vi "PMS7003_read_v2_subVi.vi"(8 "error in (no error)":errorcluster, 10 "UART connected":bool, 11 "VISA Refnum in":refnum<visa-resource-name>) -> (0 "error out":errorcluster, 1 "Boolean":bool, 2 "VISA Refnum out":refnum<visa-resource-name>, 3 "output cluster":cluster{"PM1.0":i32, "PM2.5":i32, "PM10":i32})   [LabVIEW 2019]
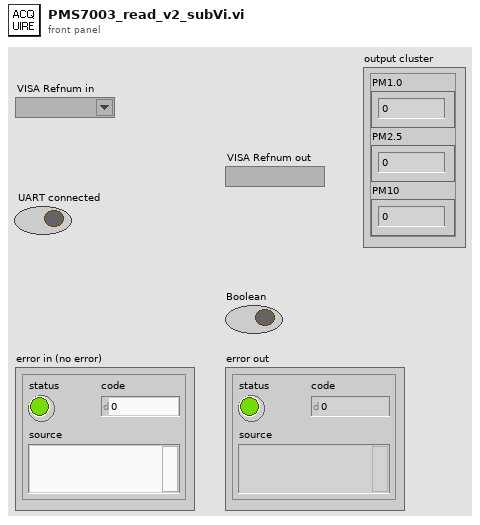
[diagram p1: front panel]
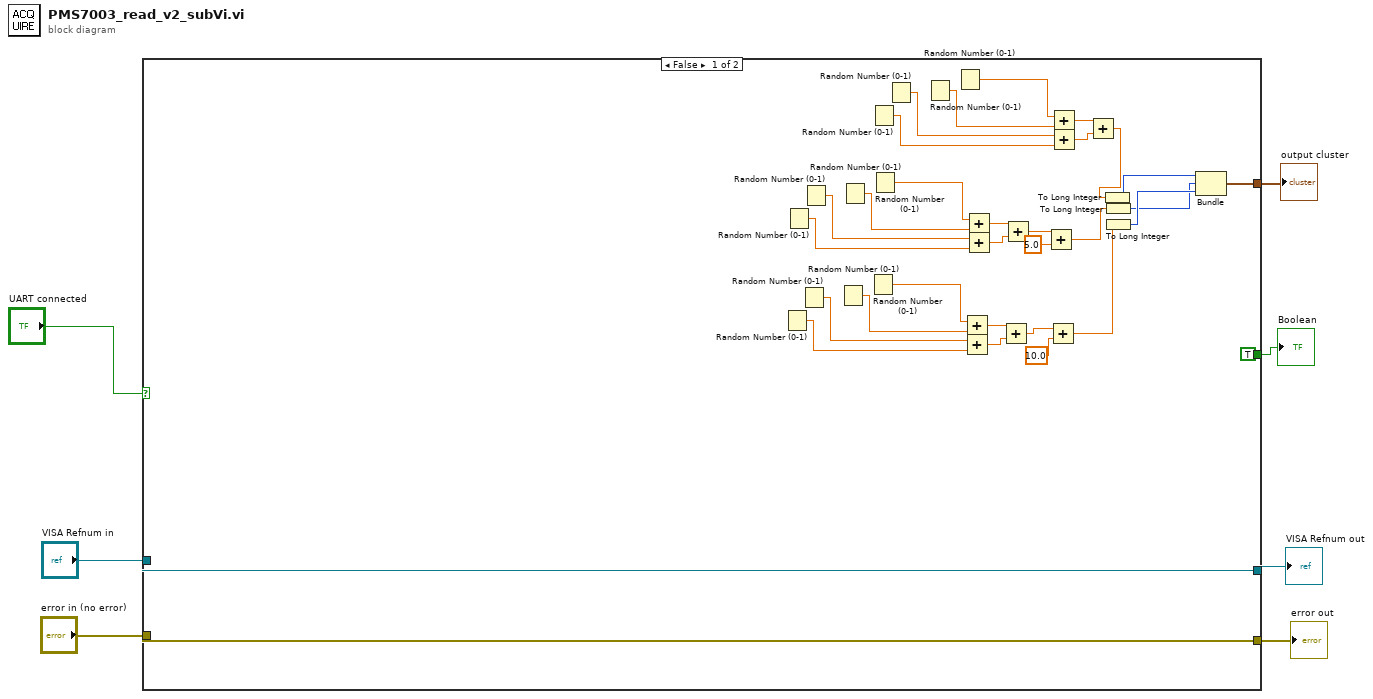
[diagram p0: block diagram]
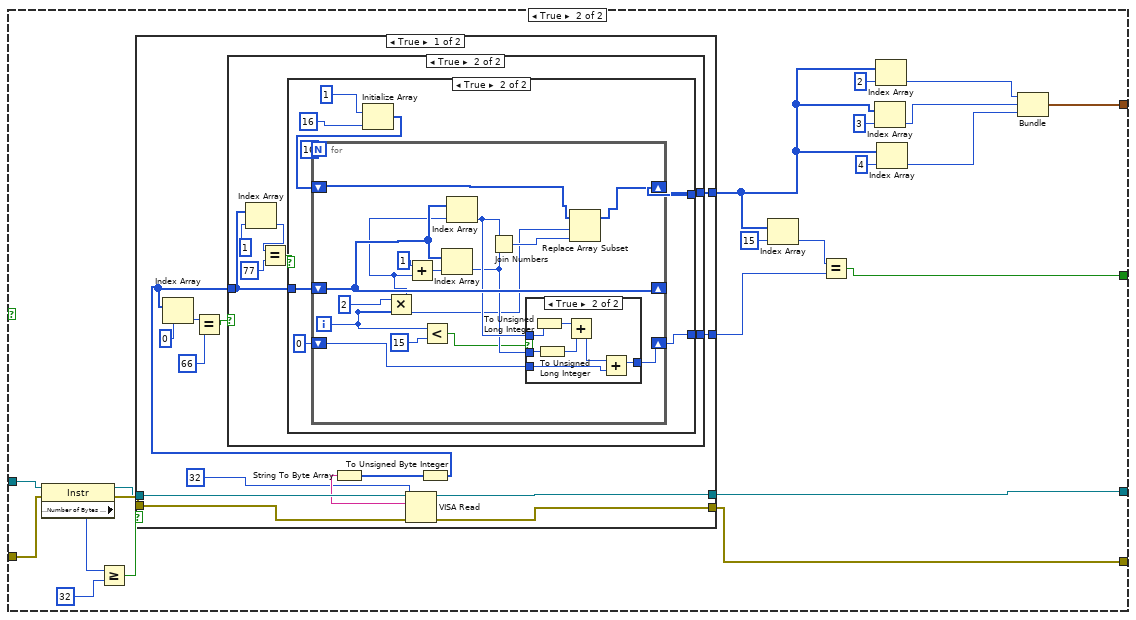
[diagram p2: hidden frame]
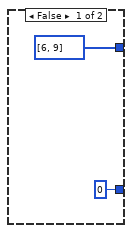
[diagram p3: hidden frame]
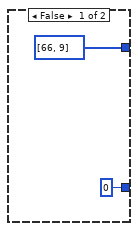
[diagram p4: hidden frame]
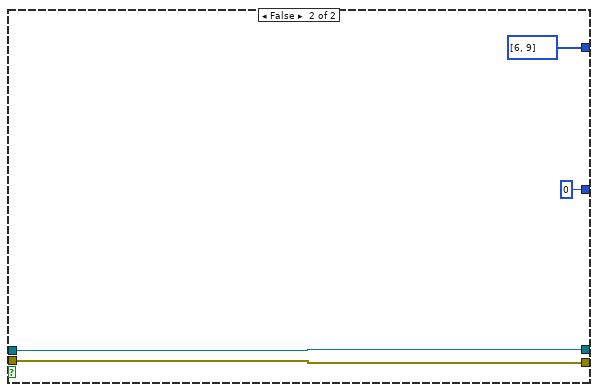
[diagram p6: hidden frame]
diagram:
  n1 = case shown="False" "UART connected" {
    tunnel: "error in (no error)" -> [w38 w59]
    tunnel: "VISA Refnum in" -> [w39 w58]
    tunnel: [TRUE w50] -> w5
    tunnel: [w39 w49] -> w3
    tunnel: [w30 w41] -> w2
    tunnel: [w38 w40] -> w1
    frame False {
      n2 = Random Number (0-1)() -> (number: 0 to 1=w20:dbl)
      n3 = Random Number (0-1)() -> (number: 0 to 1=w26:dbl)
      n4 = Random Number (0-1)() -> (number: 0 to 1=w21:dbl)
      n5 = Random Number (0-1)() -> (number: 0 to 1=w27:dbl)
      n6 = Random Number (0-1)() -> (number: 0 to 1=w22:dbl)
      n7 = Random Number (0-1)() -> (number: 0 to 1=w28:dbl)
      n8 = Random Number (0-1)() -> (number: 0 to 1=w23:dbl)
      n9 = Random Number (0-1)() -> (number: 0 to 1=w33:dbl)
      n10 = Random Number (0-1)() -> (number: 0 to 1=w29:dbl)
      n11 = Random Number (0-1)() -> (number: 0 to 1=w34:dbl)
      n12 = Random Number (0-1)() -> (number: 0 to 1=w35:dbl)
      n13 = Random Number (0-1)() -> (number: 0 to 1=w36:dbl)
      n14 = Add(x=w23, y=w22) -> (x+y=w19:dbl)
      n15 = Add(x=w21, y=w20) -> (x+y=w18:dbl)
      n16 = Add(x=w29, y=w28) -> (x+y=w25:dbl)
      n17 = Add(x=w27, y=w26) -> (x+y=w24:dbl)
      n18 = Add(x=w19, y=w18) -> (x+y=w10:dbl)
      n19 = Add(x=w25, y=w24) -> (x+y=w13:dbl)
      n20 = Add(x=w13, y=5.0) -> (x+y=w11:dbl)
      n21 = Add(x=w10, y=10.0) -> (x+y=w8:dbl)
      n22 = Add(x=w36, y=w35) -> (x+y=w32:dbl)
      n23 = Add(x=w34, y=w33) -> (x+y=w31:dbl)
      n24 = Add(x=w32, y=w31) -> (x+y=w17:dbl)
      n25 = To Long Integer(number=w17) -> (32bit integer=w14:i32)
      n26 = To Long Integer(number=w11) -> (32bit integer=w15:i32)
      n27 = To Long Integer(number=w8) -> (32bit integer=w16:i32)
      n28 = Bundle(w14, w15, w16) -> (w30:cluster{i32, i32, i32})  [unwired: 1 in]
    }
    frame True {
      n29 = property class="Instr"(reference=w58, error in=w59) -> (reference out=w54:refnum<visa-resource-name>, error out=w55:errorcluster, "Serial Settings:Number of Bytes at Serial Port"=w60:u32)
      n30 = Greater Or Equal?(x=w60, y=u32 32) -> (x >= y?=w57:bool)
      n31 = case shown="True" w57 {
        tunnel: [w72 w120] -> w49
        tunnel: w54 -> [w74 w120]
        tunnel: [w71 w119] -> w40
        tunnel: w55 -> [w73 w119]
        tunnel: [w68 u16[] [6, 9]] -> w48
        tunnel: [w62 u32 0] -> w52
        frame True {
          n32 = VISA Read(VISA resource name=w74, byte count=u32 32 ("Read Count 2"), error in (no error)=w73) -> (VISA resource name out=w72:refnum<visa-resource-name>, read buffer=w70:string, error out=w71:errorcluster)  [unwired: 1 out]
          n33 = String To Byte Array(string=w70) -> (unsigned byte array=w69:u8[])
          n34 = To Unsigned Byte Integer(number=w69) -> (unsigned 8bit integer=w63:u8[])
          n35 = Index Array(array=w63, index=0) -> (element=w66:u8)
          n36 = Equal?(x=w66, y=u8 66) -> (x = y?=w64:bool)
          n37 = case shown="True" w64 {
            tunnel: w63 -> [_ w82]
            tunnel: [u16[] [6, 9] w83] -> w68
            tunnel: [u32 0 w77] -> w62
            frame False {
            }
            frame True {
              n38 = Index Array(array=w82, index=1) -> (element=w79:u8)
              n39 = Equal?(x=w79, y=u8 77) -> (x = y?=w78:bool)
              n40 = case shown="True" w78 {
                tunnel: w82 -> [_ w93]
                tunnel: [u16[] [66, 9] w91] -> w83
                tunnel: [u32 0 w87] -> w77
                frame False {
                }
                frame True {
                  n41 = Initialize Array(1 ("index"), 16 ("index")) -> (w90:i32[])
                  n42 = for {
                    N: 16 -> [_]
                    shift-right: [w108] -> _
                    shift-left: w93 -> [w108]
                    shift-right: [w103] -> w91
                    shift-left: w90 -> [w104]
                    shift-right: [w100] -> w87
                    shift-left: u32 0 -> [w96]
                    i -> [w98]
                    n43 = Multiply(x=2, y=w98) -> (x*y=w94:i32)
                    n44 = Add(x=1, y=w94) -> (x+y=w95:i32)
                    n45 = Less?(x=w98, y=15) -> (x < y?=w99:bool)
                    n46 = Index Array(array=w108, index=w95) -> (element=w101:u8)
                    n47 = Index Array(array=w108, index=w94) -> (element=w102:u8)
                    n48 = Join Numbers(hi=w102, lo=w101) -> ((hi.lo)=w105:u16)
                    n49 = case shown="True" w99 {
                      tunnel: w102 -> [_ w112]
                      tunnel: w101 -> [_ w111]
                      tunnel: [w109 w115] -> w100
                      tunnel: w96 -> [w109 w110]
                      frame False {
                      }
                      frame True {
                        n50 = To Unsigned Long Integer(number=w112) -> (unsigned 32bit integer=w113:u32)
                        n51 = To Unsigned Long Integer(number=w111) -> (unsigned 32bit integer=w114:u32)
                        n52 = Add(x=w113, y=w114) -> (x+y=w116:u32)
                        n53 = Add(x=w116, y=w110) -> (x+y=w115:u32)
                      }
                    }
                    n54 = Replace Array Subset(array=w104, new element=w105, index=w98) -> (w103:i32[])
                  }
                }
              }
            }
          }
        }
        frame False {
        }
      }
      n55 = Index Array(array=w48, index=15) -> (element=w53:i32)
      n56 = Equal?(x=w53, y=w52) -> (x = y?=w50:bool)
      n57 = Index Array(array=w48, index=3) -> (element=w43:i32)
      n58 = Index Array(array=w48, index=2) -> (element=w42:i32)
      n59 = Index Array(array=w48, index=4) -> (element=w44:i32)
      n60 = Bundle("index"=w42, "index"=w43, "index"=w44) -> (w41:cluster{"index":i32, "index":i32, "index":i32})  [unwired: 1 in]
    }
  }
  "Boolean" <- w5
  "VISA Refnum out" <- w3
  "output cluster" <- w2
  "error out" <- w1
